vi "PH_Timing.evt call Set PU Delay.vi"(0 "i ref in":refnum<vi>, 1 "Instance":string="N/A", 2 "Power Unit":string, 3 "Delay":dbl, 5 "error in (no error)":errorcluster) -> (14 "i ref out":refnum<vi>, 19 "error out":errorcluster)   [LabVIEW 2014, in "PH_Timing.lvlib"]
doc: "This VI sets the PU generator delay by a simple call."
uses:
  PH_Timing.lvlib
  CSCore/CSSystem/CoreLib/CoreLib.string 2 byte array.vi
  CSCore/CSSystem/CoreLib/CoreLib.double 2 byte array.vi
  CSCore/CSSystem/CoreLib/CoreLib.lvlib
  CSCore/BaseProcess/BaseProcess.lvlib
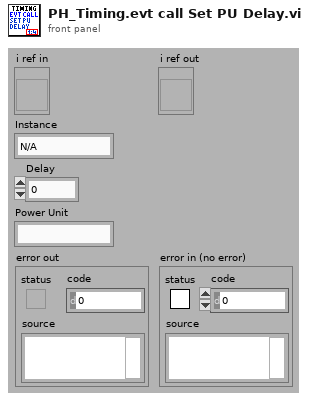
[diagram p1: front panel]
types:
  T1 = typedef "CoreDefs.rawDataType.ctl" = i8[]
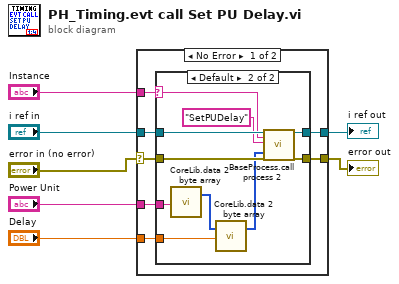
[diagram p0: block diagram]
diagram:
  n1 = case shown="No Error" "error in (no error)" {
    selector: "error in (no error)" -> [w11 w28]
    tunnel: [w14 w27] -> w7
    tunnel: [w13 w28] -> w6
    tunnel: "i ref in" -> [w12 w27]
    tunnel: "Instance" -> [w10 _]
    tunnel: "Power Unit" -> [w9 _]
    tunnel: "Delay" -> [w8 _]
    frame No Error {
      n2 = case shown="Default" w10 {
        selector: w10 -> [_ w21]
        tunnel: [w16 w26] -> w14
        tunnel: [w15 w25] -> w13
        tunnel: w12 -> [w16 w24]
        tunnel: w11 -> [w15 w22]
        tunnel: w9 -> [_ w18]
        tunnel: w8 -> [_ w20]
        frame "N/A" {
        }
        frame Default {
          n3 = call-poly "CoreLib.data 2 byte array.vi"("string"=w18) -> ("byteArray out"=w19:T1)  [unwired: 18 in]
          n4 = call-poly "CoreLib.data 2 byte array.vi"("byteArray"=w19, "f64"=w20) -> ("byteArray out"=w17:T1)  [unwired: 17 in]
          n5 = call "BaseProcess.call process 2.vi"("i ref in"=w24, "Object"=w21, "Selector"="SetPUDelay", "Data"=w17, "error in (no error)"=w22) -> ("i ref out"=w26:refnum<vi>, "error out"=w25:errorcluster)  [unwired: 13 in]
        }
      }
    }
    frame Error {
    }
  }
  "error out" <- w6
  "i ref out" <- w7
